vi "Message to Byte Array.vi"(0 "Input Data":T1 {"Command" format="%02x"; "Destination" format="%02x"; "Source" format="%02x"}, 11 "Error In":errorcluster) -> (4 "Byte Array":u8[](array[numeric]), 15 "Error Out":errorcluster)   [LabVIEW 2023]
uses:
  type defs/Data In.ctl
  D:/Common/LabVIEW GEA2 Toolkit/source/GEA3 DLL Source/Utilities.dll
  source/GEA3 DLL Source/Utilities.dll
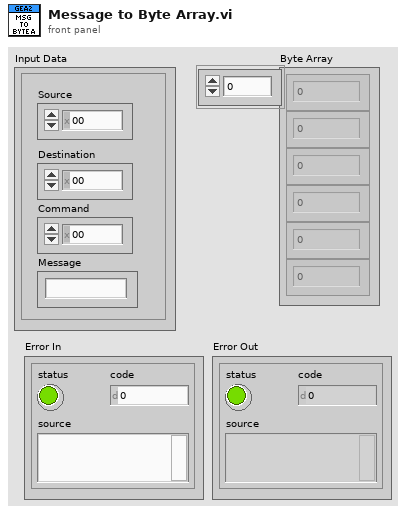
[diagram p1: front panel]
types:
  T1 = typedef "Data In.ctl" = cluster{"Source":u8, "Destination":u8, "Command":u8, "Message":string}
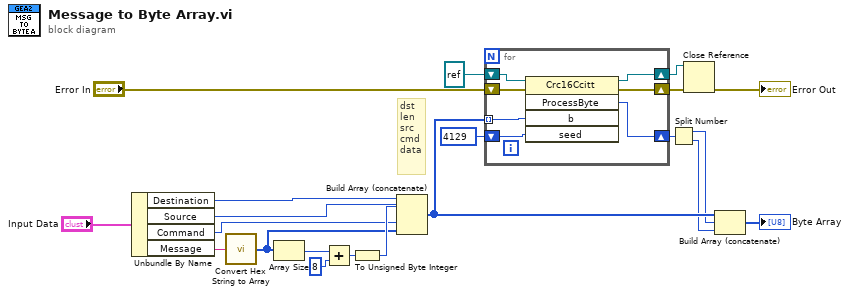
[diagram p0: block diagram]
diagram:
  # "dst\nlen\nsrc\ncmd\ndata"
  n1 = Unbundle By Name("Input Data") -> ("Destination"=w4:u8, "Source"=w3:u8, "Command"=w2:u8, "Message"=w1:string)
  n2 = call "Convert Hex String to Array.vi"("Hex String In"=w1) -> ("Hex Array Out"=w16:u8[])  [unwired: 14 in]
  n3 = Array Size(array=w16) -> (size(s)=w17:i32)
  n4 = Add(x=w17, y=8) -> (x+y=w20:i32)
  n5 = To Unsigned Byte Integer(number=w20) -> (unsigned 8bit integer=w19:u8)
  n6 = Build Array (concatenate)(w4, w19, w3, w2, w16) -> (w8:u8[])
  n7 = for {
    tunnel: w8 -> [w28] mode=indexing
    shift-right: [w26] -> w14
    shift-left: u16 4129 ("seed") -> [w27]
    shift-right: [w24] -> w12
    shift-left: "Error In" -> [w25]
    shift-right: [w22] -> w11
    shift-left: refnum<k24> refnum ("reference") -> [w23]
    n8 = invoke class="Crc16Ccitt" method="ProcessByte"(reference=w23, error in=w25, "b"=w28, "seed"=w27) -> (reference out=w22:refnum<k24>, error out=w24:errorcluster, "ProcessByte"=w26:u16)  [unwired: 1 in, 2 out]
  }
  n9 = Split Number(x=w14) -> (hi(x)=w6:u8, lo(x)=w7:u8)
  n10 = Close Reference(reference=w11, error in (no error)=w12) -> (error out=→"Error Out":errorcluster)
  n11 = Build Array (concatenate)(w8, w6, w7) -> (→"Byte Array":u8[])
